vi "Command_Joint_Velocity.vi"(0 "Side":T1, 1 "node":string, 2 "Arm Velocities":T2, 3 "error in":errorcluster) -> (6 "error out":errorcluster)   [LabVIEW 2013]
uses:
  ROS/Code/SubVIs/BaxterArmsSmall.ctl
  ROS/Code/SubVIs/BaxterSide.ctl
panel:
  out "Move Command":string
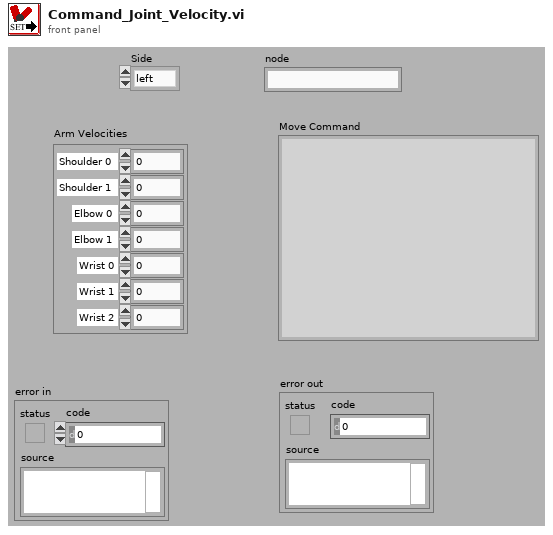
[diagram p1: front panel]
types:
  T1 = typedef "BaxterSide.ctl" = enum16{"left", "right"}
  T2 = typedef "BaxterArmsSmall.ctl" = cluster{"Elbow 0":dbl, "Elbow 1":dbl, "Shoulder 0":dbl, "Shoulder 1":dbl, "Wrist 0":dbl, "Wrist 1":dbl, "Wrist 2":dbl}
  T3 = typedef "_ROSControl.ctl" = cluster{"topic port":u16, "Node":string, "topic":string, "type":string, "node port":u32, "error ":errorcluster, "Direction":T4, "APIs":string[]}
  T4 = typedef "_ROSDirection.ctl" = enum16{"Node", "Publisher", "Subscriber", "Service Client"}
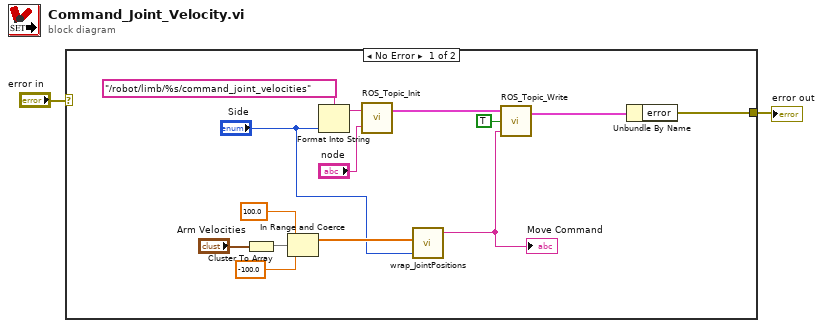
[diagram p0: block diagram]
diagram:
  n1 = case shown="No Error" "error in" {
    selector: "error in" -> [_ w17]
    tunnel: [w11 w17] -> w2
    frame No Error {
      n2 = Cluster To Array(cluster="Arm Velocities") -> (array=w10:dbl[])
      n3 = In Range and Coerce(upper limit=100.0 ("Elbow 0"), x=w10, lower limit=-100.0 ("Elbow 0")) -> (coerced(x)=w8:dbl[])  [unwired: 1 out]
      n4 = Format Into String(format string="/robot/limb/%s/command_joint_velocities" ("topic"), "Side") -> (resulting string=w13:string)  [unwired: 2 in, 1 out]
      n5 = call "ROS_Topic_Init.vi"("node"="node", "topic"=w13) -> ("ROS out"=w12:T3)  [unwired: 1 in]
      n6 = call "wrap_JointPositions.vi"("Side"="Side", "Positions"=w8) -> ("msg out"=w6:string)  [unwired: 3 in]
      "Move Command" <- w6
      n7 = call "ROS_Topic_Write.vi"("Msg in"=w6, "Continuous?"=TRUE, "ROS in"=w12) -> ("ROS out"=w15:T3)  [unwired: 1 in]
      n8 = Unbundle By Name(w15) -> ("error"=w11:errorcluster)
    }
    frame Error {
    }
  }
  "error out" <- w2
